vi "MultiScale Pyramids LL SubVI.vi"(8 "error in (no error)":errorcluster, 10 "Image Dst":T1, 11 "Image Src":T1) -> (0 "error out":errorcluster, 3 "Image Dst Out":T1)   [LabVIEW 2023]
uses:
  Conv Flt Presets.ctl
  <vilib>/vision/Image Controls.llb/IMAQ Image.ctl
  <vilib>/vision/NI_Vision_Development_Module.lvlib
panel:
  out "Pyr Levels":i32
  in  "Filters":T2[](array[typedef])=[enum."Seifert 7x7", enum."Seifert 5x5", enum."Highlight Details 3x3", enum."None", enum."None", enum."None", enum."None", enum."None", enum."None", enum."None", enum."None", enum."None"]
  in  "Threshold":sgl=30.0
  in  "Radius":sgl=33.0
  in  "Amount":sgl=6.0
  in  "Operator":u16(ring)=6 items=["Linear", "Log", "Exp", "Square", "Square root", "Power X", "Power 1/X"]
  in  "X Value":sgl=1.2 format="%.2f"
  in  "LUT Multiplier":sgl[](array[slide])=[157.53847, 185.1077, 192.98462, 248.12308, 196.92308, 248.12308, 252.06154, 114.215385, 248.12308, 110.276924, 102.4, 102.4] scale=0.0..512.0
  in  "LUT Power":sgl[](array[slide])=[0.61538464, 0.43076923, 0.3846154, 0.43846154, 0.42307693, 0.5538462, 0.64615387, 0.61538464, 0.61538464, 0.6, 0.4, 0.4] scale=0.0..2.0
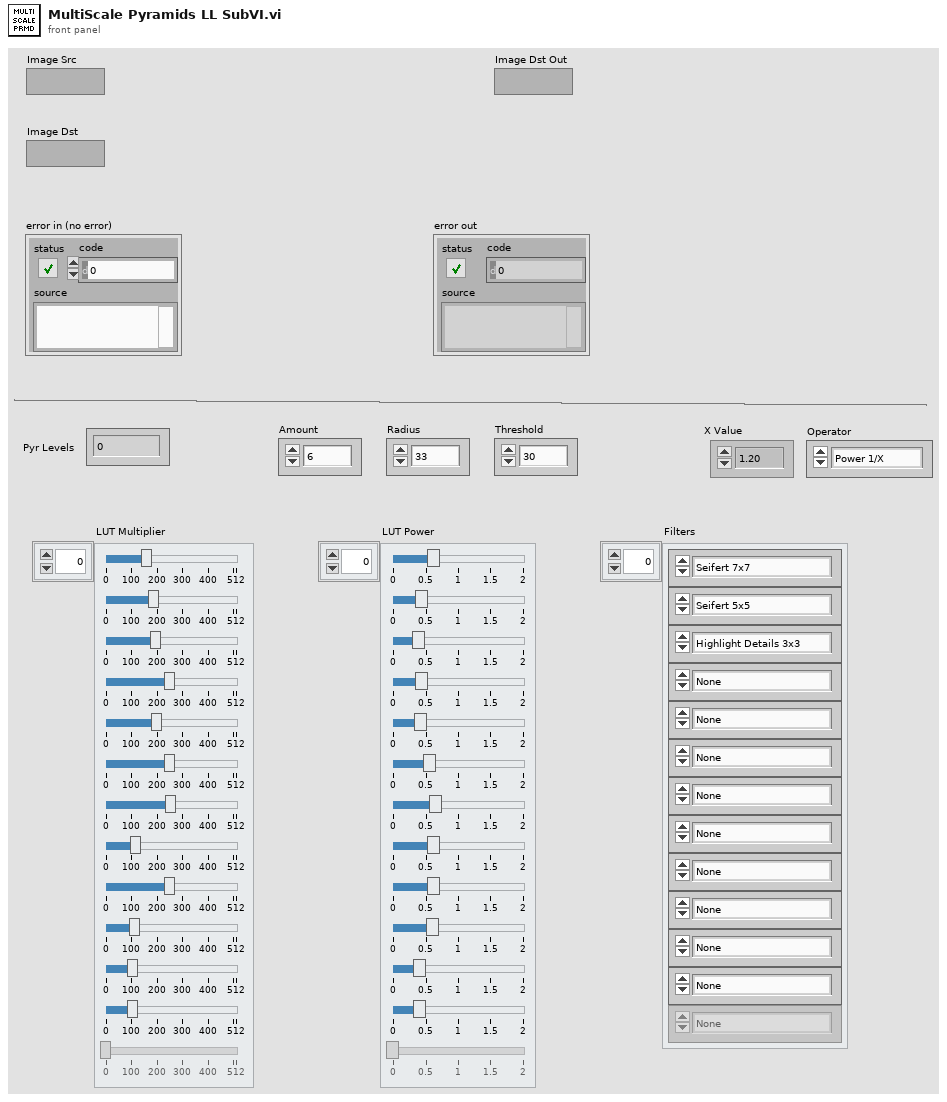
[diagram p1: front panel]
types:
  T1 = typedef "IMAQ Image.ctl" = refnum<image>
  T2 = typedef "Conv Flt Presets.ctl" = enum16{"None", "Seifert 5x5", "Seifert 7x7", "High Pass 5x5 ", "High Pass 7x7", "Highlight Details 3x3", "Highlight Details 5x5", "Highlight Detail 7x7"}
  T3 = typedef "Image Type" = u32
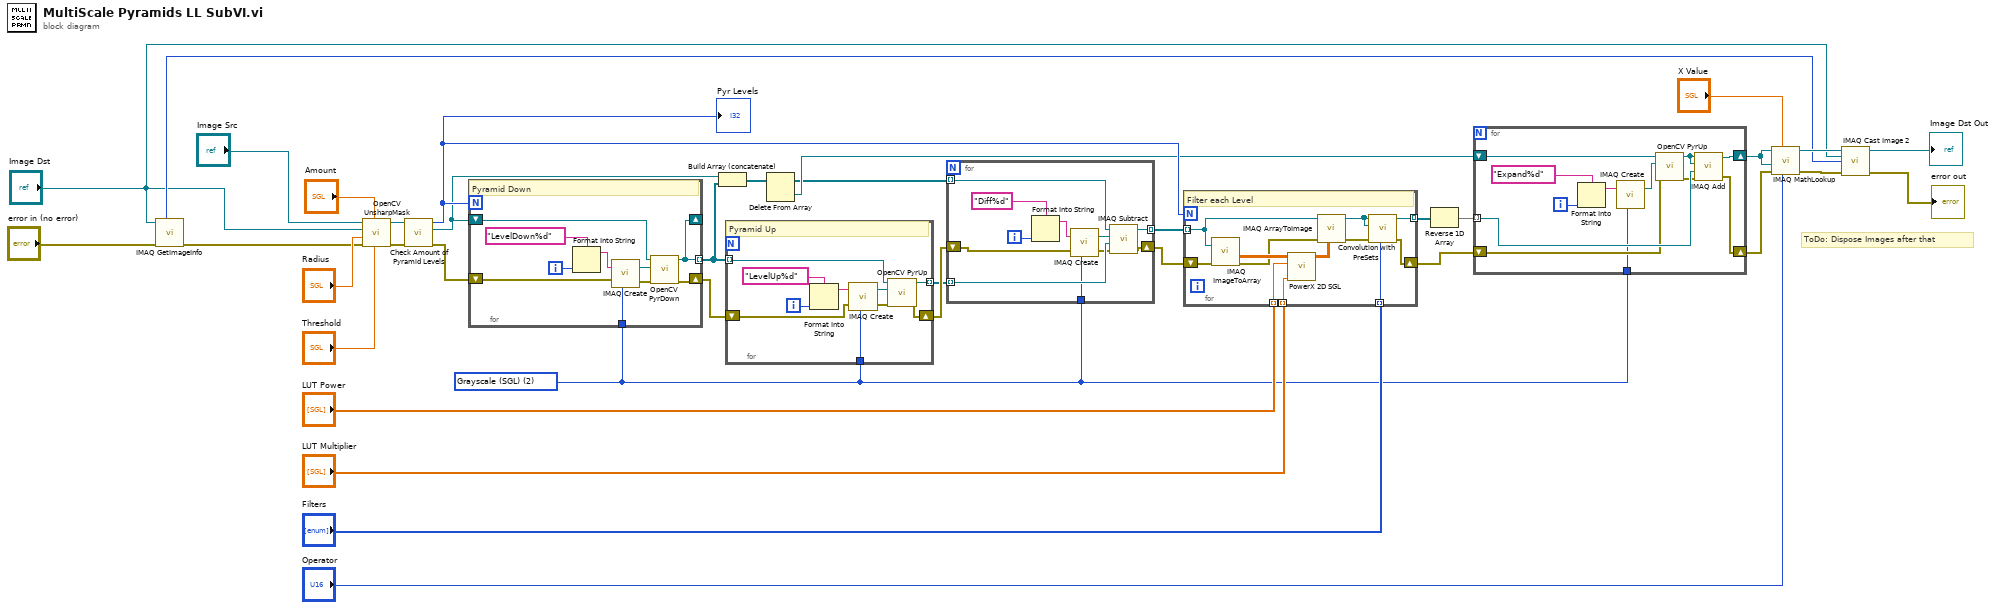
[diagram p0: block diagram]
diagram:
  w1 = T3 2 items=["Grayscale (U8)", "Grayscale (I16)", "Grayscale (SGL)", "Complex (CSG)", "RGB (U32)", "HSL (U32)", "RGB (U64)", "Grayscale (U16)"] ("Image Type")
  # "ToDo: Dispose Images after that"
  n1 = call "IMAQ GetImageInfo"("error in (no error)"="error in (no error)", "Image"="Image Dst") -> ("error out"=w2:errorcluster, "Image Type"=w5:T3)  [unwired: 2 in, 6 out]
  n2 = call "OpenCV UnsharpMask.vi"("Threshold"="Threshold", "Amount"="Amount", "error in (no error)"=w2, "Radius"="Radius", "Image Dst"="Image Dst", "Image Src"="Image Src") -> ("error out"=w33:errorcluster, "Image Dst Out"=w35:T1)  [unwired: 4 in]
  n3 = call "Check Amount of Pyramid Levels.vi"("error in (no error)"=w33, "Refnum in"=w35) -> ("error out"=w34:errorcluster, "Image Dup"=w36:T1, "Pyr Levels"=w37:i32)  [unwired: 7 in]
  "Pyr Levels" <- w37
  n4 = for {
    N: w37 -> [_]
    shift-right: [w43] -> _
    shift-left: w36 -> [w45]
    tunnel: [w43] -> w23 mode=indexing
    shift-right: [w39] -> w26
    shift-left: w34 -> [w41]
    tunnel: w1 -> [w38]
    i -> [w42]
    # "Pyramid Down"
    n5 = Format Into String(format string="LevelDown%d", w42) -> (resulting string=w46:string)  [unwired: 2 in, 1 out]
    n6 = call "IMAQ Create"("Image Name"=w46, "Image Type"=w38, "error in (no error)"=w41) -> ("New Image"=w44:T1, "error out"=w40:errorcluster)  [unwired: 2 in]
    n7 = call "OpenCV PyrDown.vi"("error in (no error)"=w40, "Image Dst"=w44, "Image Src"=w45) -> ("error out"=w39:errorcluster, "Image Dst Out"=w43:T1)  [unwired: 7 in]
  }
  n8 = Build Array (concatenate)(w36, w23) -> (w6:T1[])
  n9 = for {
    tunnel: [w54] -> w8 mode=indexing
    tunnel: w23 -> [w53] mode=indexing
    shift-right: [w49] -> w27
    shift-left: w26 -> [w51]
    tunnel: w1 -> [w48]
    i -> [w52]
    # "Pyramid Up"
    n10 = Format Into String(format string="LevelUp%d", w52) -> (resulting string=w56:string)  [unwired: 2 in, 1 out]
    n11 = call "IMAQ Create"("Image Name"=w56, "Image Type"=w48, "error in (no error)"=w51) -> ("New Image"=w55:T1, "error out"=w50:errorcluster)  [unwired: 2 in]
    n12 = call "OpenCV PyrUp.vi"("error in (no error)"=w50, "Image Dst"=w55, "Image Src"=w53) -> ("error out"=w49:errorcluster, "Image Dst Out"=w54:T1)  [unwired: 7 in]
  }
  n13 = Delete From Array(array=w6) -> (deleted portion=w9:T1, array with subset deleted=w7:T1[])  [unwired: 2 in]
  n14 = for {
    tunnel: w7 -> [w65] mode=indexing
    tunnel: w8 -> [w64] mode=indexing
    tunnel: [w62] -> w14 mode=indexing
    shift-right: [w59] -> w28
    shift-left: w27 -> [w61]
    tunnel: w1 -> [w58]
    i -> [w66]
    n15 = Format Into String(format string="Diff%d", w66) -> (resulting string=w68:string)  [unwired: 2 in, 1 out]
    n16 = call "IMAQ Create"("Image Name"=w68, "Image Type"=w58, "error in (no error)"=w61) -> ("New Image"=w63:T1, "error out"=w60:errorcluster)  [unwired: 2 in]
    n17 = call "IMAQ Subtract"("Image Src A"=w65, "Image Dst"=w63, "Image Src B"=w64, "error in (no error)"=w60) -> ("Image Dst Out"=w62:T1, "error out"=w59:errorcluster)  [unwired: 3 in]
  }
  n18 = for {
    N: w37 -> [_]
    tunnel: w14 -> [w80] mode=indexing
    tunnel: [w79] -> w11 mode=indexing
    tunnel: "LUT Power" -> [w75] mode=indexing
    tunnel: "LUT Multiplier" -> [w74] mode=indexing
    tunnel: "Filters" -> [w73] mode=indexing
    shift-right: [w69] -> w29
    shift-left: w28 -> [w70]
    # "Filter each Level"
    n19 = call "IMAQ ImageToArray"("error in (no error)"=w70, "Image"=w80) -> ("Image Pixels (Float)"=w77:sgl[][], "error out"=w72:errorcluster)  [unwired: 2 in, 3 out]
    n20 = call "PowerX 2D SGL.vi"("Multiplier"=w74, "Power"=w75, "Signal In"=w77) -> ("Signal Out"=w76:sgl[][])  [unwired: 8 in]
    n21 = call "IMAQ ArrayToImage"("Image Pixels (Float)"=w76, "error in (no error)"=w72, "Image"=w80) -> ("error out"=w71:errorcluster, "Image Out"=w78:T1)  [unwired: 7 in]
    n22 = call "Convolution with PreSets.vi"("Filter"=w73, "error in (no error)"=w71, "Image Dst"=w78, "Image Src"=w78) -> ("error out"=w69:errorcluster, "Image Dst Out"=w79:T1)  [unwired: 5 in, 1 out]
  }
  n23 = Reverse 1D Array(array=w11) -> (reversed array=w10:T1[])
  n24 = for {
    shift-right: [w85] -> w17
    shift-left: w9 -> [w88]
    tunnel: w10 -> [w86] mode=indexing
    shift-right: [w82] -> w30
    shift-left: w29 -> [w84]
    tunnel: w1 -> [w81]
    i -> [w89]
    n25 = Format Into String(format string="Expand%d", w89) -> (resulting string=w91:string)  [unwired: 2 in, 1 out]
    n26 = call "IMAQ Create"("Image Name"=w91, "Image Type"=w81) -> ("New Image"=w90:T1)  [unwired: 3 in, 1 out]
    n27 = call "OpenCV PyrUp.vi"("error in (no error)"=w84, "Image Dst"=w90, "Image Src"=w88) -> ("error out"=w83:errorcluster, "Image Dst Out"=w87:T1)  [unwired: 7 in]
    n28 = call "IMAQ Add"("Image Src A"=w87, "Image Dst"=w87, "Image Src B"=w86, "error in (no error)"=w83) -> ("Image Dst Out"=w85:T1, "error out"=w82:errorcluster)  [unwired: 3 in]
  }
  n29 = call "IMAQ MathLookup"("Operator"="Operator", "X Value"="X Value", "error in (no error)"=w30, "Image Dst"=w17, "Image Src"=w17) -> ("error out"=w31:errorcluster, "Image Dst Out"=w16:T1)  [unwired: 5 in]
  n30 = call "IMAQ Cast Image 2"("Image Src"=w16, "Image Dst"="Image Dst", "Image Type"=w5, "error in (no error)"=w31) -> ("Image Dst Out"=→"Image Dst Out":T1, "error out"=→"error out":errorcluster)  [unwired: 10 in]
